vi "Cluster-Unbundle & Bundle [By Name].vi"() -> ()   [LabVIEW 2016]
panel:
  in  "Cluster 3":T1
  out "Cluster 2":T1
  out "Boolean":bool
  out "String":string
  out "Numeric":dbl
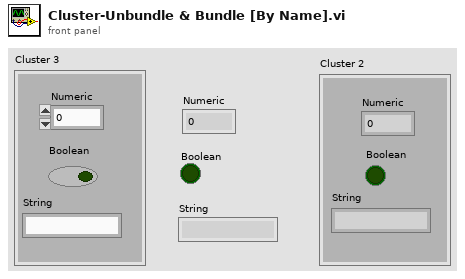
[diagram p1: front panel]
types:
  T1 = cluster{"Numeric":dbl, "Boolean":bool, "String":string}
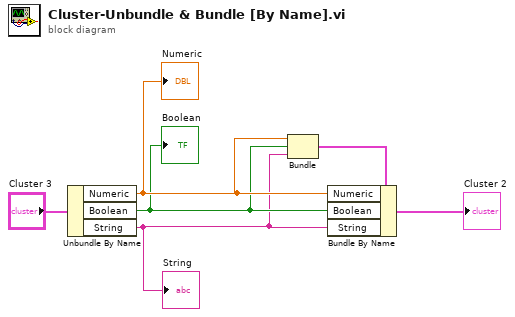
[diagram p0: block diagram]
diagram:
  n1 = Unbundle By Name("Cluster 3") -> ("Numeric"=w4:dbl, "Boolean"=w3:bool, "String"=w2:string)
  "Numeric" <- w4
  "String" <- w2
  "Boolean" <- w3
  n2 = Bundle("Numeric"=w4, "Boolean"=w3, "String"=w2) -> (w1:T1)  [unwired: 1 in]
  n3 = Bundle By Name(cluster=w1, "Numeric"=w4, "Boolean"=w3, "String"=w2) -> (→"Cluster 2":T1)
